vi "ControlProperty.vi"() -> ()   [LabVIEW 2016]
panel:
  in  "Visible ?":bool
  in  "Disabled":T1(ring)
  in  "Numeric":dbl
  in  "OK":bool
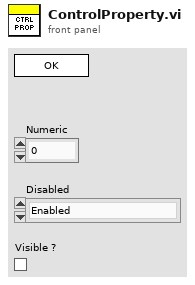
[diagram p1: front panel]
types:
  T1 = enum8{"Enabled", "Disabled", "Disabled and Grayed Out"}
  T2 = enum32{"Invalid", "Standard", "Closed", "Hidden", "Minimized", "Maximized"}
  T3 = enum32{"invalid app kind", "Development System", "Run Time System", "Student Edition", "Embedded LabVIEW", "Evaluation", "Custom"}
  T4 = cluster{"Core":cluster{"Current VI Reference":refnum<vi>, "Close Panel on Exit?":bool}, "Your Boolean data":bool, "Your string data":string}
  T5 = cluster{"Current VI Reference":refnum<vi>, "Close Panel on Exit?":bool}
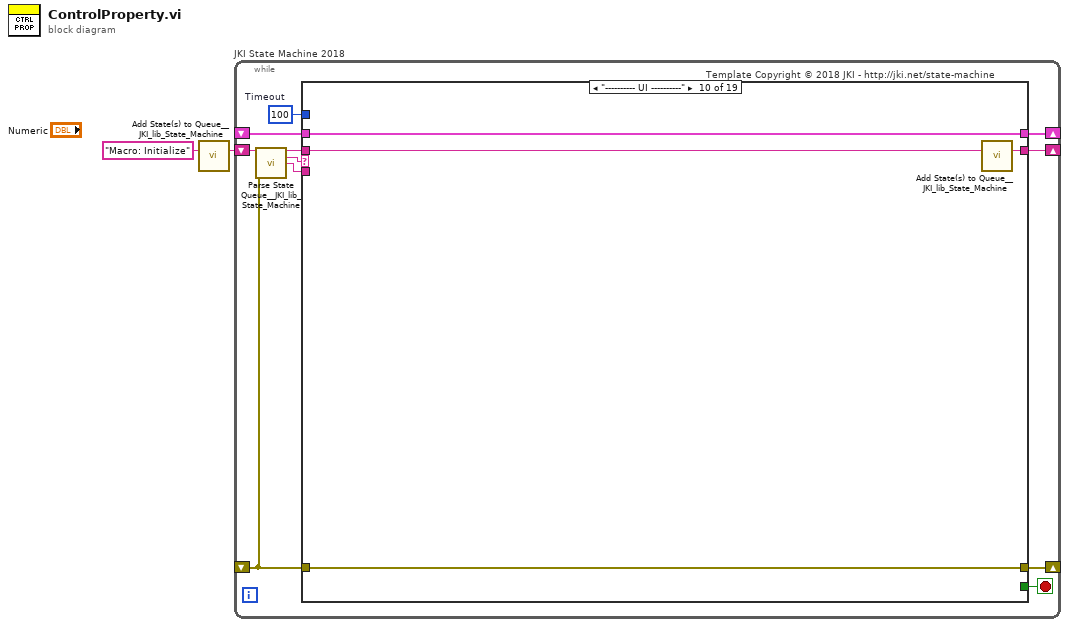
[diagram p0: block diagram]
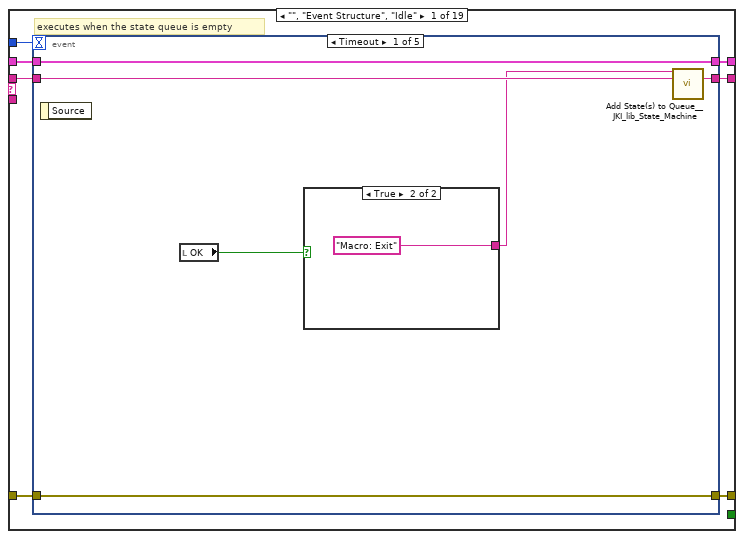
[diagram p2: hidden frame]
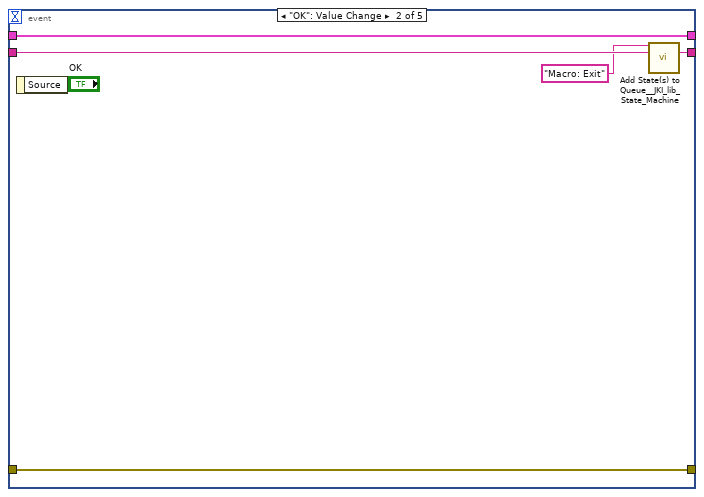
[diagram p4: hidden frame]
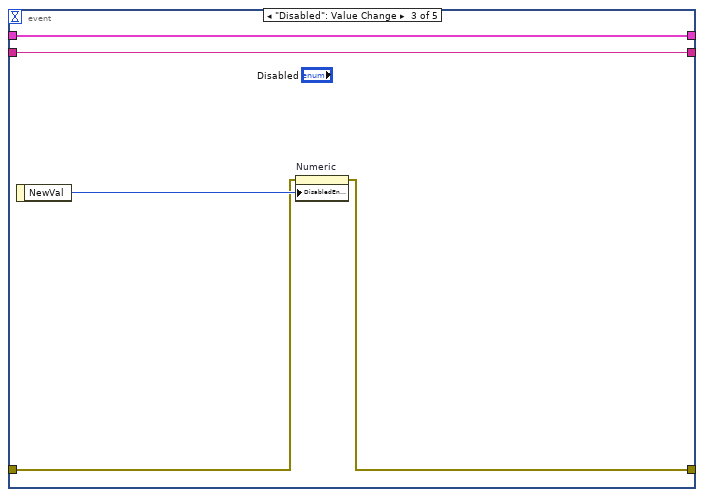
[diagram p5: hidden frame]
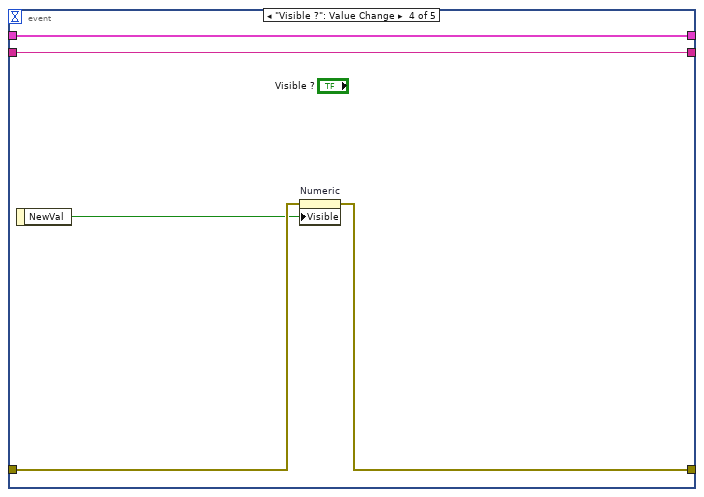
[diagram p6: hidden frame]
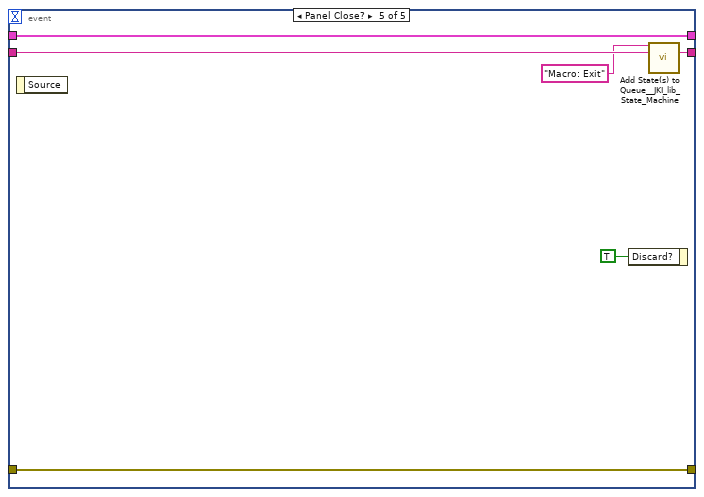
[diagram p7: hidden frame]
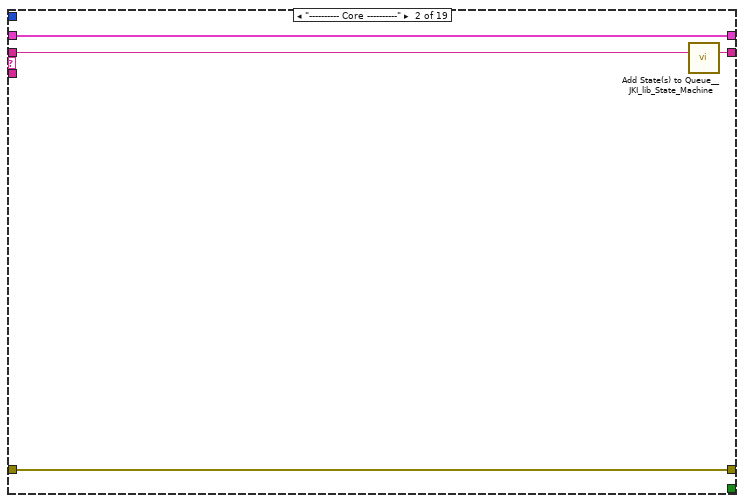
[diagram p8: hidden frame]
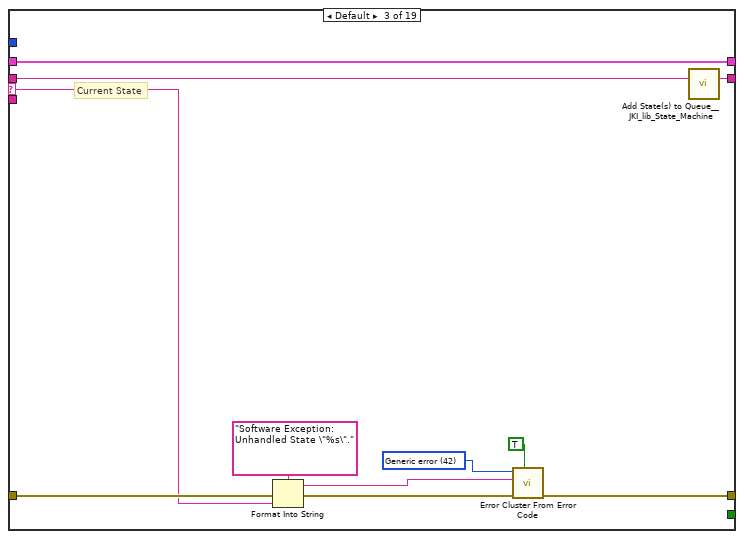
[diagram p9: hidden frame]
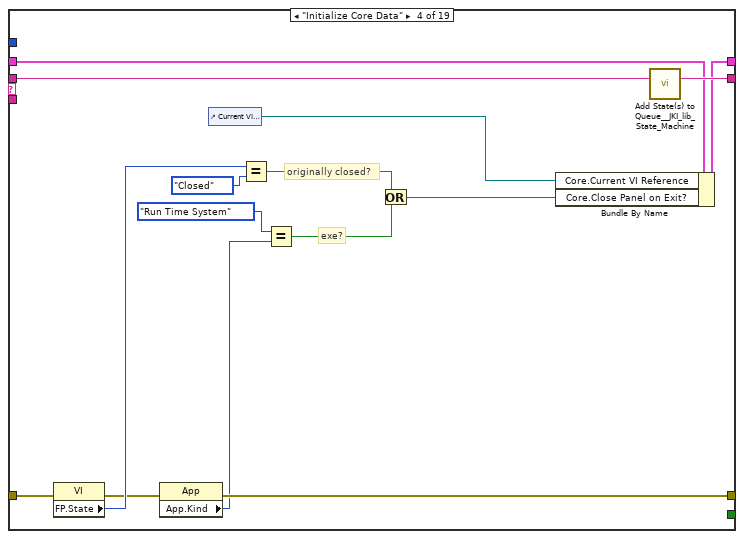
[diagram p10: hidden frame]
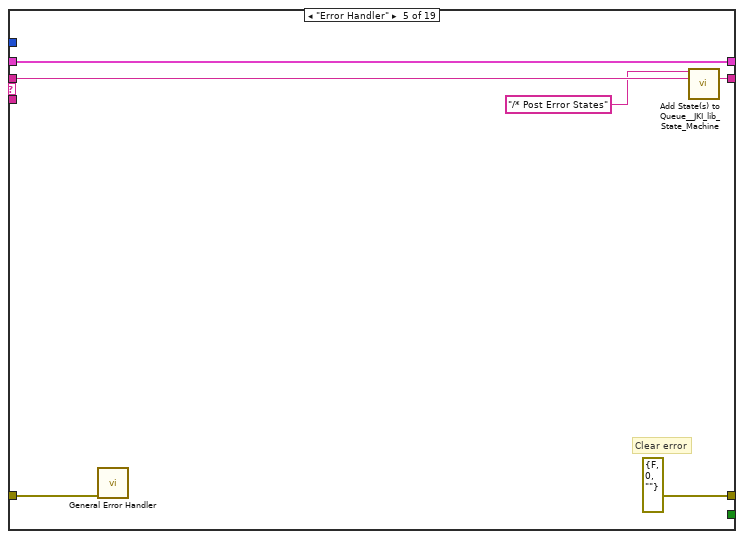
[diagram p11: hidden frame]
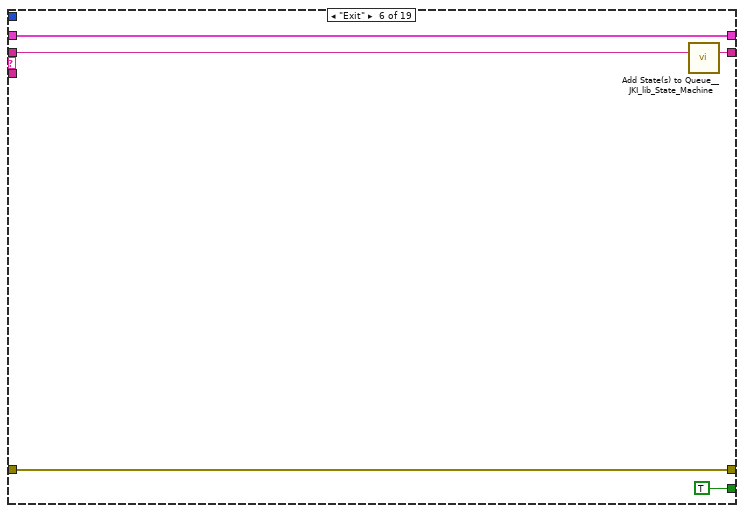
[diagram p12: hidden frame]
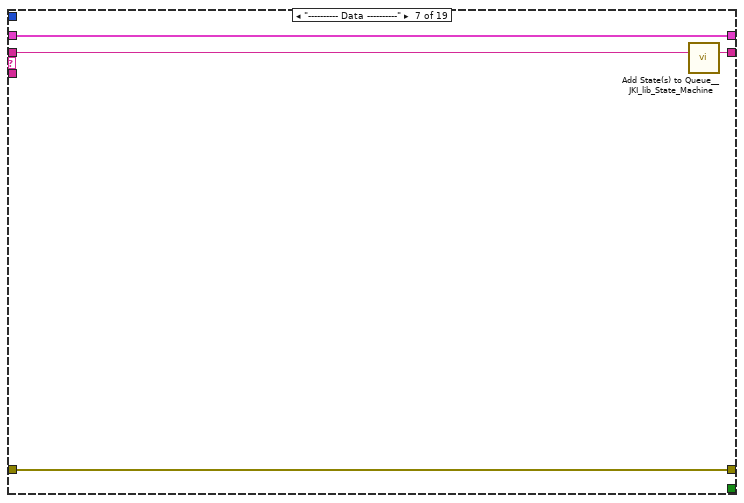
[diagram p13: hidden frame]
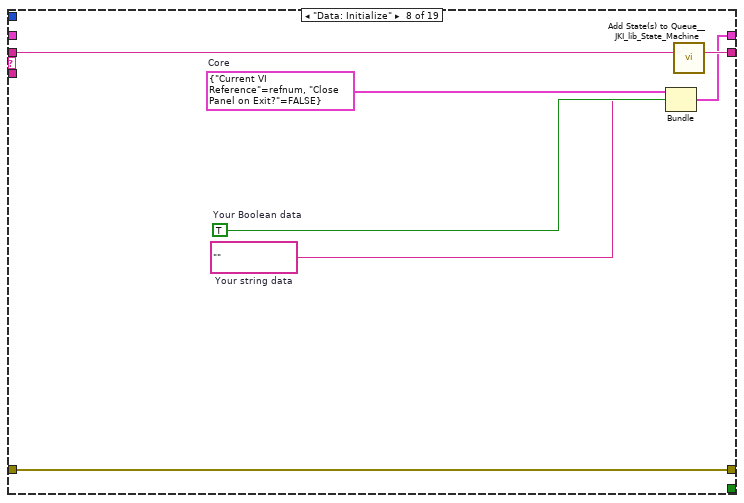
[diagram p14: hidden frame]
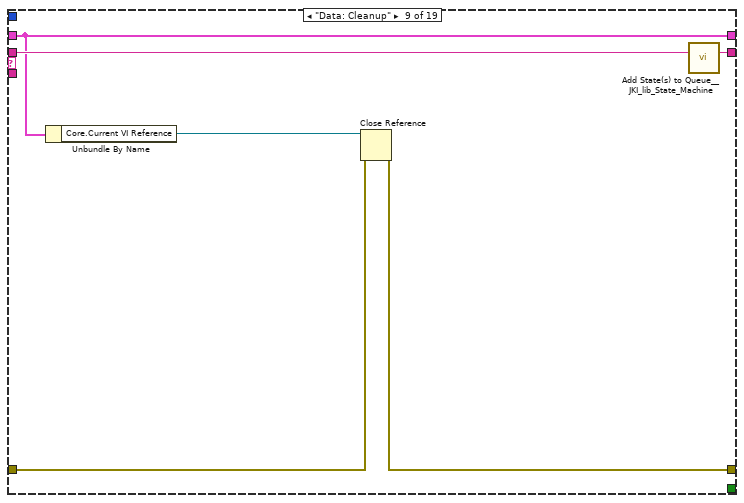
[diagram p15: hidden frame]
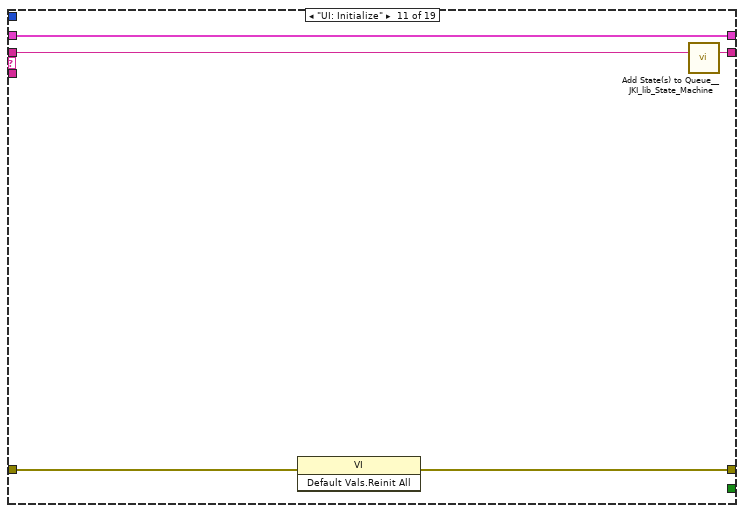
[diagram p16: hidden frame]
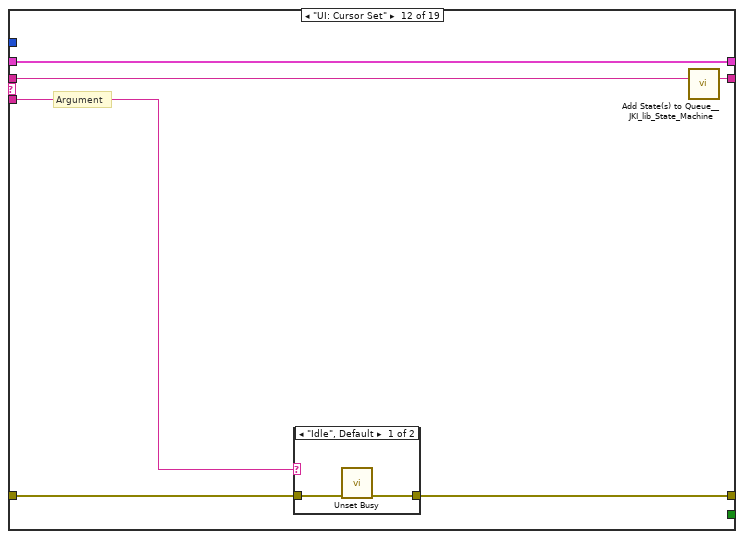
[diagram p17: hidden frame]
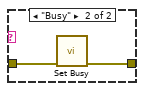
[diagram p18: hidden frame]
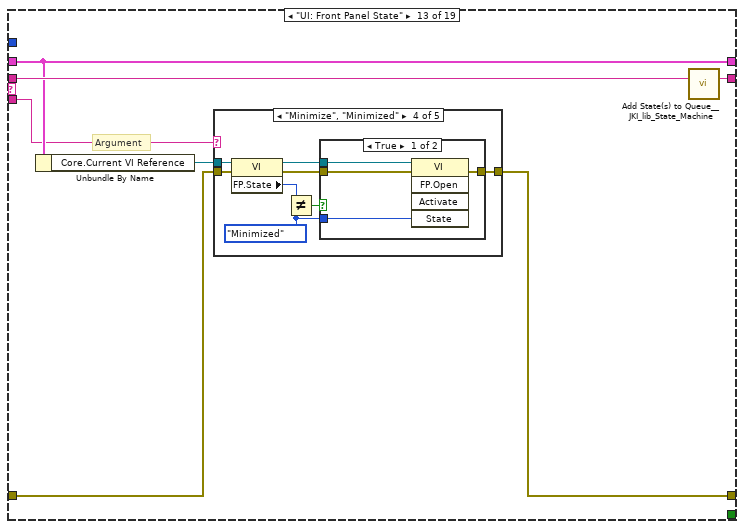
[diagram p19: hidden frame]
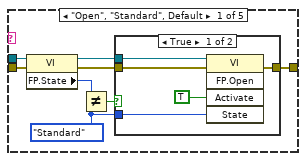
[diagram p20: hidden frame]
diagram:
  n1 = call <vilib>:"Add State(s) to Queue__JKI_lib_State_Machine.vi"("State(s) in (\"\")"="Macro: Initialize") -> ("States Out"=w2:string)  [unwired: 14 in]
  n2 = while "JKI State Machine 2018" {
    shift-right: [w6] -> _
    shift-left: _ -> [w5]
    shift-right: [w9] -> _
    shift-left: _ -> [w3]
    shift-right: [w8] -> _
    shift-left: w2 -> [w10]
    stop <- w7 stop-if-true
    w4 = 100  # Timeout
    # "Template Copyright © 2018 JKI - http://jki.net/state-machine"
    n3 = call <vilib>:"Parse State Queue__JKI_lib_State_Machine.vi"("State Queue"=w10, "Error In (no error)"=w3) -> ("Remaining States"=w12:string, "Current State"=w13:string, "Arguments"=w11:string)  [unwired: 11 in]
    n4 = case shown="\"---------- UI ----------\"" w13 {
      selector: w13 -> [_ _ w53 _ _ _ _ _ _ _ _ _ _ _ _ _ _ _ _]
      tunnel: w12 -> [w20 w52 w57 w78 w84 w89 w93 w100 w106 w110 w115 w121 w132 w201 w206 w216 w220 w224 w228]
      tunnel: w11 -> [_ _ _ _ _ _ _ _ _ _ _ w116 w126 _ _ _ _ _ _]
      tunnel: w5 -> [w18 w49 w55 w74 w81 w87 w90 _ w101 w107 w113 w119 w128 w198 w203 w213 w217 w221 w225]
      tunnel: [w17 w50 w59 w66 errorcluster {"status"=FALSE, "code"=0, "source"=""} ("error out") w86 w91 w97 w102 w108 w111 w117 w129 w199 w204 w214 w218 w222 w226] -> w9
      tunnel: w3 -> [w16 w50 w58 w68 w80 w86 w91 w97 w103 w108 w112 w118 w130 w199 w204 w214 w218 w222 w226]
      tunnel: [w19 w51 w56 w77 w83 w88 w92 w99 w105 w109 w114 w120 w131 w200 w205 w215 w219 w223 w227] -> w8
      tunnel: [_ _ _ _ _ TRUE _ _ _ _ _ _ _ _ _ _ _ _ _] -> w7
      tunnel: [w15 w49 w55 w76 w81 w87 w90 w98 w101 w107 w113 w119 w128 w198 w203 w213 w217 w221 w225] -> w6
      tunnel: w4 -> [w14 _ _ _ _ _ _ _ _ _ _ _ _ _ _ _ _ _ _]
      frame "", "Event Structure", "Idle" {
        # "executes when the state queue is empty"
        n5 = event shown="[0] Timeout" {
          selector: _ -> [_ _ _ _ _]
          dyn-events: _ -> [_ _ _ _ _]
          timeout: w14 -> [_ _ _ _ _]
          tunnel: w20 -> [w26 w32 w37 w42 w48]
          tunnel: [w25 w31 w37 w42 w47] -> w19
          tunnel: w18 -> [w23 w29 w36 w41 w45]
          tunnel: [w24 w30 w33 w39 w46] -> w17
          tunnel: w16 -> [w24 w30 w34 w40 w46]
          tunnel: [w23 w29 w36 w41 w45] -> w15
          event Timeout {
            n6 = event-data() -> ()  [unwired: 1 in, 1 out]
            n7 = local read "OK"() -> (w21:bool)
            n8 = case shown="True" w21 {
              tunnel: [_ "Macro: Exit"] -> w22
              frame False {
              }
              frame True {
              }
            }
            n9 = call <vilib>:"Add State(s) to Queue__JKI_lib_State_Machine.vi"("State(s) in Front (\"\")"=w22, "State(s) in (\"\")"=w26) -> ("States Out"=w25:string)  [unwired: 13 in]
          }
          event "OK": Value Change {
            n10 = event-data() -> ()  [unwired: 1 in, 1 out]
            n11 = call <vilib>:"Add State(s) to Queue__JKI_lib_State_Machine.vi"("State(s) in Front (\"\")"="Macro: Exit", "State(s) in (\"\")"=w32) -> ("States Out"=w31:string)  [unwired: 13 in]
          }
          event "Disabled": Value Change {
            n12 = event-data() -> ("NewVal"=w35:T1)  [unwired: 1 in]
            n13 = property on="Numeric" class="DigNum (strict)"(error in=w34, "DisabledEnum"=w35) -> (error out=w33:errorcluster)  [unwired: 1 in, 1 out]
          }
          event "Visible ?": Value Change {
            n14 = event-data() -> ("NewVal"=w38:bool)  [unwired: 1 in]
            n15 = property on="Numeric" class="DigNum (strict)"(error in=w40, "Visible"=w38) -> (error out=w39:errorcluster)  [unwired: 1 in, 1 out]
          }
          event Panel Close? {
            n16 = event-data() -> ()  [unwired: 1 in, 1 out]
            n17 = event-data("Discard?"=TRUE) -> ()  [unwired: 1 in, 1 out]
            n18 = call <vilib>:"Add State(s) to Queue__JKI_lib_State_Machine.vi"("State(s) in Front (\"\")"="Macro: Exit", "State(s) in (\"\")"=w48) -> ("States Out"=w47:string)  [unwired: 13 in]
          }
        }
      }
      frame "---------- Core ----------" {
        n19 = call <vilib>:"Add State(s) to Queue__JKI_lib_State_Machine.vi"("State(s) in (\"\")"=w52) -> ("States Out"=w51:string)  [unwired: 14 in]
      }
      frame Default {
        w62 = 42 items=["No error", "Argument error", "Memory is full", "Out of zone", "End of file", "File already open", "Generic file I/O error", "File not found", "File permission error", "Disk is full", "Duplicate path", "Too many files open", "System feature not enabled", "Resource file not found", "Cannot add resource", "Resource not found", "Image not found", "Image memory error", "Pen does not exist", "Config type invalid", "Config token not found", "Config parse error", "Config memory error", "Bad external code format", "Bad external code offset", "External code not present", "Null window", "Destroy window error", "Null menu", "Print aborted", "Bad print record", "Print driver error", "Windows error during printing", "Memory error during printing", "Print dialog error", "Generic print error", "Invalid device refnum", "Device not found", "Device parameter error", "Device unit error", "Cannot open device", "Device call aborted", "Generic error", "Cancelled by user", "Object ID too low", "Object ID too high", "Object not in heap", "Unknown heap", "Unknown object (invalid DefProc)", "Unknown object (DefProc not in table)", "Message out of range", "Invalid (null) method", "Unknown message", "Manager call not supported", "Bad address", "Network operation in progress", "Network operation timed out", "Connection is busy", "Network attribute not supported", "Network error", "Address in use", "System out of memory", "Connection aborted", "Connection refused", "Not connected", "Already connected", "Connection closed", "Initialization error (interapplication manager)", "Bad occurrence", "Wait on unbound occurrence handler", "Occurrence queue overflow", "Datalog type conflict", "Unused", "Unrecognized type (interapplication manager)", "Memory corrupt", "Failed to make temporary DLL", "Old CIN version", "Drag socket not found", "Failed to load drop-object", "Failed to register OLE object", "Failed to release OLE object", "Format specifier type mismatch", "Unknown format specifier", "Too few format specifiers", "Too many format specifiers", "Scan failed", "Newer CIN version", "Error converting to variant", "Runtime menu error", "Password tampered", "Variant attribute not found", "Incompatible variant data type", "Event data is not available", "Event Store is not present", "Occurrence is not found", "Event Queue is not created", "Event info is not available", "Refnum passed is NULL", "Error retrieving Class GUID", "Error retrieving CoClass GUID", "Error retrieving TypeLib GUID.", "Bad built application magic bytes.", "Specific driver is different from the specific driver associated with the Logical Name.", "There is no session opened to the class driver.", "Max Error", "MAX - Error with config objects", "MAX - Error loading configuration", "MAX - Group not supported"]
        # "Current State"
        n20 = Format Into String(format string="Software Exception: Unhandled State \"%s\"." ("message"), error in=w58, w53) -> (resulting string=w61:string, error out=w60:errorcluster)  [unwired: 1 in]
        n21 = call <vilib>:"Error Cluster From Error Code.vi"("show call chain? (False)"=TRUE, "error in (no error)"=w60, "error message (\"\")"=w61, "error code (0)"=w62) -> ("error out"=w59:errorcluster)  [unwired: 5 in]
        n22 = call <vilib>:"Add State(s) to Queue__JKI_lib_State_Machine.vi"("State(s) in (\"\")"=w57) -> ("States Out"=w56:string)  [unwired: 14 in]
      }
      frame "Initialize Core Data" {
        # "originally closed?"
        # "exe?"
        n23 = property class="VI"(error in=w68) -> (error out=w67:errorcluster, "FP.State"=w71:T2)  [unwired: 1 in, 1 out]
        n24 = property class="App"(error in=w67) -> (error out=w66:errorcluster, "App.Kind"=w64:T3)  [unwired: 1 in, 1 out]
        n25 = control-ref of="Current VI Reference"() -> (w72:refnum<vi>)
        n26 = Equal?(x=w71, y=T2."Closed" ("Front Panel Window:State")) -> (x = y?=w69:bool)
        n27 = Equal?(x=T3."Run Time System" ("Application:Kind"), y=w64) -> (x = y?=w75:bool)
        n28 = Or(x=w69, y=w75) -> (x .or. y?=w73:bool)
        n29 = Bundle By Name(cluster=w74, "Core.Current VI Reference"=w72, "Core.Close Panel on Exit?"=w73) -> (w76:T4)
        n30 = call <vilib>:"Add State(s) to Queue__JKI_lib_State_Machine.vi"("State(s) in (\"\")"=w78) -> ("States Out"=w77:string)  [unwired: 14 in]
      }
      frame "Error Handler" {
        # "Clear error"
        n31 = call <vilib>:"General Error Handler.vi"("error in (no error)"=w80) -> ()  [unwired: 10 in, 5 out]
        n32 = call <vilib>:"Add State(s) to Queue__JKI_lib_State_Machine.vi"("State(s) in Front (\"\")"="/* Post Error States", "State(s) in (\"\")"=w84) -> ("States Out"=w83:string)  [unwired: 13 in]
      }
      frame "Exit" {
        n33 = call <vilib>:"Add State(s) to Queue__JKI_lib_State_Machine.vi"("State(s) in (\"\")"=w89) -> ("States Out"=w88:string)  [unwired: 14 in]
      }
      frame "---------- Data ----------" {
        n34 = call <vilib>:"Add State(s) to Queue__JKI_lib_State_Machine.vi"("State(s) in (\"\")"=w93) -> ("States Out"=w92:string)  [unwired: 14 in]
      }
      frame "Data: Initialize" {
        w94 = T5 {"Current VI Reference"=refnum, "Close Panel on Exit?"=FALSE}  # Core
        w96 = TRUE  # Your Boolean data
        w95 = ""  # Your string data
        n35 = Bundle("Core"=w94, "Your Boolean data"=w96, "Your string data"=w95) -> (w98:T4)  [unwired: 1 in]
        n36 = call <vilib>:"Add State(s) to Queue__JKI_lib_State_Machine.vi"("State(s) in (\"\")"=w100) -> ("States Out"=w99:string)  [unwired: 14 in]
      }
      frame "Data: Cleanup" {
        n37 = Unbundle By Name(w101) -> ("Core.Current VI Reference"=w104:refnum<vi>)
        n38 = Close Reference(reference=w104, error in (no error)=w103) -> (error out=w102:errorcluster)
        n39 = call <vilib>:"Add State(s) to Queue__JKI_lib_State_Machine.vi"("State(s) in (\"\")"=w106) -> ("States Out"=w105:string)  [unwired: 14 in]
      }
      frame "---------- UI ----------" {
        n40 = call <vilib>:"Add State(s) to Queue__JKI_lib_State_Machine.vi"("State(s) in (\"\")"=w110) -> ("States Out"=w109:string)  [unwired: 14 in]
      }
      frame "UI: Initialize" {
        n41 = invoke class="VI" method="Default Vals.Reinit All"(error in=w112) -> (error out=w111:errorcluster)  [unwired: 2 in, 2 out]
        n42 = call <vilib>:"Add State(s) to Queue__JKI_lib_State_Machine.vi"("State(s) in (\"\")"=w115) -> ("States Out"=w114:string)  [unwired: 14 in]
      }
      frame "UI: Cursor Set" {
        # "Argument"
        n43 = case shown="\"Idle\", Default" w116 {
          tunnel: w118 -> [w123 w125]
          tunnel: [w122 w124] -> w117
          frame "Idle", Default {
            n44 = call <vilib>:"Unset Busy.vi"("error in (no error)"=w123) -> ("error out"=w122:errorcluster)  [unwired: 10 in]
          }
          frame "Busy" {
            n45 = call <vilib>:"Set Busy.vi"("error in (no error)"=w125) -> ("error out"=w124:errorcluster)  [unwired: 9 in, 1 out]
          }
        }
        n46 = call <vilib>:"Add State(s) to Queue__JKI_lib_State_Machine.vi"("State(s) in (\"\")"=w121) -> ("States Out"=w120:string)  [unwired: 14 in]
      }
      frame "UI: Front Panel State" {
        # "Argument"
        n47 = Unbundle By Name(w128) -> ("Core.Current VI Reference"=w127:refnum<vi>)
        n48 = case shown="\"Minimize\", \"Minimized\"" w126 {
          tunnel: w130 -> [w138 w153 w164 w177 w190]
          tunnel: [w140 w154 w166 w179 w192] -> w129
          tunnel: w127 -> [w139 w151 w165 w178 w191]
          frame "Open", "Standard", Default {
            w133 = T2."Standard" ("State")
            n49 = property class="VI"(reference=w139, error in=w138) -> (reference out=w136:refnum<vi>, error out=w137:errorcluster, "FP.State"=w135:T2)
            n50 = Not Equal?(x=w135, y=w133) -> (x != y?=w134:bool)
            n51 = case shown="True" w134 {
              tunnel: [w144 w146] -> w140
              tunnel: w137 -> [w143 w146]
              tunnel: w136 -> [w142 _]
              tunnel: w133 -> [w141 _]
              frame True {
                n52 = invoke class="VI" method="FP.Open"(reference=w142, error in=w143, "Activate"=TRUE, "State"=w141) -> (error out=w144:errorcluster)  [unwired: 1 in, 4 out]
              }
              frame False {
              }
            }
          }
          frame "Close", "Closed" {
            n53 = property class="VI"(reference=w151, error in=w153) -> (reference out=w150:refnum<vi>, error out=w152:errorcluster, "FP.State"=w148:T2)
            n54 = Not Equal?(x=w148, y=T2."Closed" ("Front Panel Window:State")) -> (x != y?=w147:bool)
            n55 = case shown="True" w147 {
              tunnel: [w155 w158] -> w154
              tunnel: w152 -> [w155 w157]
              tunnel: w150 -> [_ w156]
              frame False {
              }
              frame True {
                n56 = invoke class="VI" method="FP.Close"(reference=w156, error in=w157) -> (error out=w158:errorcluster)  [unwired: 1 in, 2 out]
              }
            }
          }
          frame "Hidden", "Hide" {
            w159 = T2."Hidden" ("State")
            n57 = property class="VI"(reference=w165, error in=w164) -> (reference out=w162:refnum<vi>, error out=w163:errorcluster, "FP.State"=w161:T2)
            n58 = Not Equal?(x=w161, y=w159) -> (x != y?=w160:bool)
            n59 = case shown="True" w160 {
              tunnel: [w170 w171] -> w166
              tunnel: w163 -> [w169 w171]
              tunnel: w162 -> [w168 _]
              tunnel: w159 -> [w167 _]
              frame True {
                n60 = invoke class="VI" method="FP.Open"(reference=w168, error in=w169, "State"=w167) -> (error out=w170:errorcluster)  [unwired: 2 in, 4 out]
              }
              frame False {
              }
            }
          }
          frame "Minimize", "Minimized" {
            w172 = T2."Minimized" ("State")
            n61 = property class="VI"(reference=w178, error in=w177) -> (reference out=w175:refnum<vi>, error out=w176:errorcluster, "FP.State"=w174:T2)
            n62 = Not Equal?(x=w174, y=w172) -> (x != y?=w173:bool)
            n63 = case shown="True" w173 {
              tunnel: [w183 w184] -> w179
              tunnel: w176 -> [w182 w184]
              tunnel: w175 -> [w181 _]
              tunnel: w172 -> [w180 _]
              frame True {
                n64 = invoke class="VI" method="FP.Open"(reference=w181, error in=w182, "State"=w180) -> (error out=w183:errorcluster)  [unwired: 2 in, 4 out]
              }
              frame False {
              }
            }
          }
          frame "Maximize", "Maximized" {
            w185 = T2."Maximized" ("State")
            n65 = property class="VI"(reference=w191, error in=w190) -> (reference out=w188:refnum<vi>, error out=w189:errorcluster, "FP.State"=w187:T2)
            n66 = Not Equal?(x=w187, y=w185) -> (x != y?=w186:bool)
            n67 = case shown="True" w186 {
              tunnel: [w196 w197] -> w192
              tunnel: w189 -> [w195 w197]
              tunnel: w188 -> [w194 _]
              tunnel: w185 -> [w193 _]
              frame True {
                n68 = invoke class="VI" method="FP.Open"(reference=w194, error in=w195, "State"=w193) -> (error out=w196:errorcluster)  [unwired: 2 in, 4 out]
              }
              frame False {
              }
            }
          }
        }
        n69 = call <vilib>:"Add State(s) to Queue__JKI_lib_State_Machine.vi"("State(s) in (\"\")"=w132) -> ("States Out"=w131:string)  [unwired: 14 in]
      }
      frame "---------- Macro ----------" {
        n70 = call <vilib>:"Add State(s) to Queue__JKI_lib_State_Machine.vi"("State(s) in (\"\")"=w201) -> ("States Out"=w200:string)  [unwired: 14 in]
      }
      frame "Macro: Initialize" {
        w202 = "Data: Initialize\nInitialize Core Data\nUI: Initialize\nUI: Front Panel State >> Open"  # Data: Initialize Initialize Core Data UI: Initialize UI: Front Panel State >> Open
        n71 = call <vilib>:"Add State(s) to Queue__JKI_lib_State_Machine.vi"("State(s) in Front (\"\")"=w202, "State(s) in (\"\")"=w206) -> ("States Out"=w205:string)  [unwired: 13 in]
      }
      frame "Macro: Exit" {
        n72 = Unbundle By Name(w213) -> ("Core.Close Panel on Exit?"=w212:bool)
        n73 = Select(t="UI: Front Panel State >> Close", s=w212, f="") -> (s? t:f=w209:string)
        n74 = call <vilib>:"Add State(s) to Queue__JKI_lib_State_Machine.vi"("State(s) in (\"\")"=w209, "State(s) at Back (\"\")"="Data: Cleanup\nExit") -> ("States Out"=w207:string)  [unwired: 13 in]
        n75 = call <vilib>:"Add State(s) to Queue__JKI_lib_State_Machine.vi"("State(s) in Front (\"\")"=w207, "State(s) in (\"\")"=w216) -> ("States Out"=w215:string)  [unwired: 13 in]
      }
      frame "---------- New Category ----------" {
        n76 = call <vilib>:"Add State(s) to Queue__JKI_lib_State_Machine.vi"("State(s) in (\"\")"=w220) -> ("States Out"=w219:string)  [unwired: 14 in]
      }
      frame "New Category: 1" {
        n77 = call <vilib>:"Add State(s) to Queue__JKI_lib_State_Machine.vi"("State(s) in (\"\")"=w224) -> ("States Out"=w223:string)  [unwired: 14 in]
      }
      frame "New Category: 2" {
        n78 = call <vilib>:"Add State(s) to Queue__JKI_lib_State_Machine.vi"("State(s) in (\"\")"=w228) -> ("States Out"=w227:string)  [unwired: 14 in]
      }
    }
  }
